vi "Condition Get Conditions for ixScenario.vi"(8 "error in (no error)":errorcluster, 10 "ixScenario (0)":i32, 11 "Connection Refnum":T3) -> (0 "error out":errorcluster, 2 "Conditions":T1[](array[typedef]), 3 "Connection Refnum":T3)   [LabVIEW 2011]
uses:
  Summitek EXT/ODBC/SQL Controls/Connection Refnum.ctl
  Condition Record.ctl
  Condition Operators.ctl
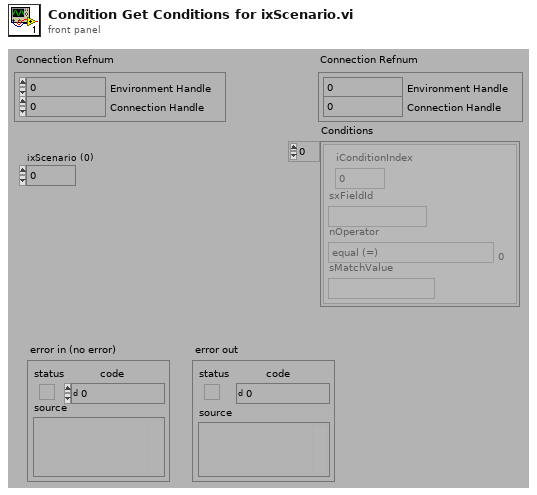
[diagram p1: front panel]
types:
  T1 = typedef "Condition Record.ctl" = cluster{"iConditionIndex":i32, "sxFieldId":string, "nOperator":T2, "sMatchValue":string}
  T2 = typedef "Condition Operators.ctl" = enum16{"equal (=)", "not equal (\\u2260)", "less than (<)", "less than or equal (\\u2264)", "greater than (>)", "greater than or equal (\\u2265)", "contains", "does not contain"}
  T3 = typedef "Connection Refnum.ctl" = cluster{"Environment Handle":i32, "Connection Handle":i32}
  T4 = typedef "Statement Refnum.ctl" = cluster{"Statement Handle":i32, "Parameter Number":u16}
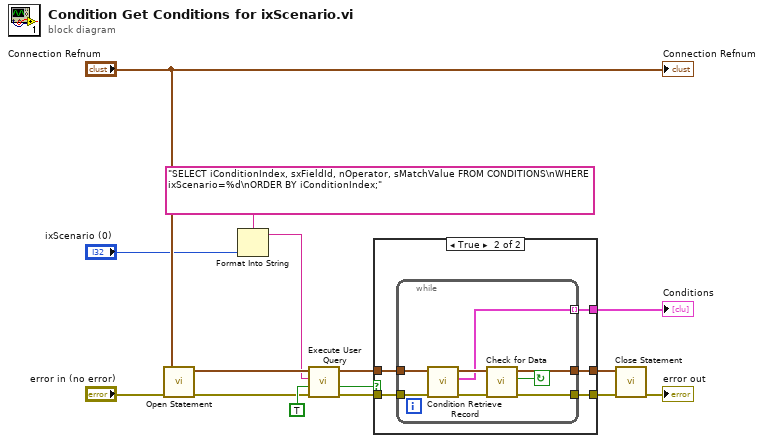
[diagram p0: block diagram]
diagram:
  n1 = call "Open Statement.vi"("error in (no error)"="error in (no error)", "Connection Refnum"="Connection Refnum") -> ("error out"=w14:errorcluster, "Statement Refnum"=w13:T4)  [unwired: 4 out]
  n2 = Format Into String(format string="SELECT iConditionIndex, sxFieldId, nOperator, sMatchValue FROM CONDITIONS\nWHERE ixScenario=%d\nORDER BY iConditionIndex;", "ixScenario (0)") -> (resulting string=w8:string)  [unwired: 2 in, 1 out]
  n3 = call "Execute User Query.vi"("error in (no error)"=w14, "Return Data? (f)"=TRUE, "User Query"=w8, "Statement Refnum"=w13) -> ("error out"=w7:errorcluster, "Data Present?"=w6:bool, "Statement Refnum"=w5:T4)  [unwired: 1 out]
  n4 = case shown="True" w6 {
    tunnel: w7 -> [w17 w20]
    tunnel: w5 -> [w16 w19]
    tunnel: [w17 w21] -> w4
    tunnel: [w16 w22] -> w3
    tunnel: [_ w18] -> w1
    frame False {
    }
    frame True {
      n5 = while {
        tunnel: [w29] -> w22
        tunnel: [w28] -> w21
        tunnel: w20 -> [w27]
        tunnel: w19 -> [w25]
        tunnel: [w23] -> w18 mode=indexing
        stop <- w30 continue-if-true
        n6 = call "Condition Retrieve Record.vi"("error in (no error)"=w27, "Statement Refnum"=w25) -> ("error out"=w26:errorcluster, "Condition"=w23:T1, "Statement Refnum"=w24:T4)  [unwired: 7 out]
        n7 = call "Check for Data.vi"("error in (no error)"=w26, "Statement Refnum"=w24) -> ("error out"=w28:errorcluster, "Data Present?"=w30:bool, "Statement Refnum"=w29:T4)  [unwired: 3 out]
      }
    }
  }
  "Conditions" <- w1
  n8 = call "Close Statement.vi"("error in (no error)"=w4, "Statement Refnum"=w3) -> ("error out"=→"error out":errorcluster)  [unwired: 5 out]
  "Connection Refnum" <- "Connection Refnum"
